vi "circ.vi"() -> ()   [LabVIEW 2009]
panel:
  in  "stop":bool
  out "Diameter 2":dbl
  out "Diameter":dbl
  out "Circumference 2":dbl
  in  "Circumference":dbl
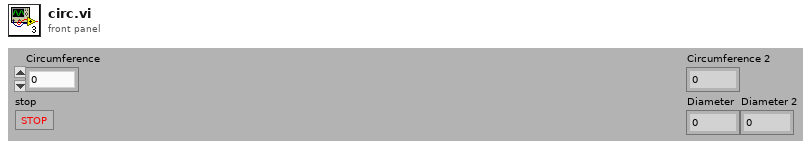
[diagram p1: front panel]
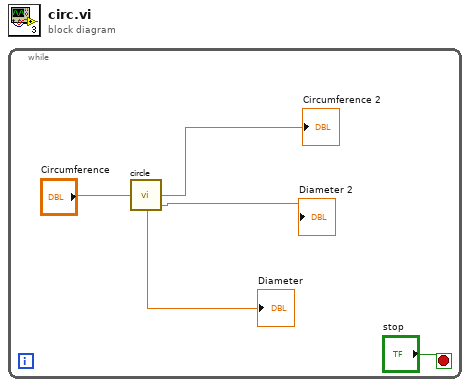
[diagram p0: block diagram]
diagram:
  n1 = while {
    stop <- "stop" stop-if-true
    n2 = call "circle.vi"("r"="Circumference") -> ("Area"=→"Diameter":dbl, "Circumference"=→"Circumference 2":dbl, "Diameter"=→"Diameter 2":dbl)
  }
